vi "Interpolate_Calib_Coeff.vi"(5 "Analysis Info cluster":T1={"Colour"=0, "Inst type"=enum."Pitot-static tube", "Inst name"="Manometer voltage", "Symbol"="U", "Code name"="", "Extra Info"="U", "Inst Array"=enum."PWA", "Index"=0, "Voltage Index"=0, "Extra Titles"=[], "Extra Values"=[]}, 6 "Calib file":path, 7 "Take New Data?":bool) -> (0 "Calib Coeff":dbl[](array[numeric]), 1 "Calib Type Name":string, 2 "Calib file string":string, 3 "Read file":bool, 4 "Analysis Info cluster  Out":T1={"Colour"=0, "Inst type"=enum."Pitot-static tube", "Inst name"="Manometer voltage", "Symbol"="U", "Code name"="", "Extra Info"="U", "Inst Array"=enum."PWA", "Index"=0, "Voltage Index"=0, "Extra Titles"=[], "Extra Values"=[]})   [LabVIEW 2010]
uses:
  Controls/Analysis_info_cluster.ctl
  Controls/Inst_type.ctl
  Controls/Instrument_Array.ctl
  XW calib map/Map method.ctl
  Globals/Meas_global.vi
  XW calib map/XW_Map_Global.vi
  Globals/Plug_in_data_global.vi
  <vilib>/Analysis/NI_AALPro.lvlib
panel:
  in  "TAKE NEW DATA XW Map method":T4=enum."Const. Psi_eff (std.)"
  in  "Domain padding factor":dbl=1.01
  in  "cap indicial sum to n":bool=TRUE
  in  "surface order (n)":i32=5
  in  "Apply calibration corrections":bool=TRUE
  in  "POST PROC. XW Map method":T4=enum."Psi_eff, k = f(Umagn.)"
  in  "variable n":bool=TRUE
  in  "wire diameter (mu.m)":dbl=5.0
  out "Header info":string[][](array[string])
  # "For polysurface method only:"
  # "For trimesh method only"
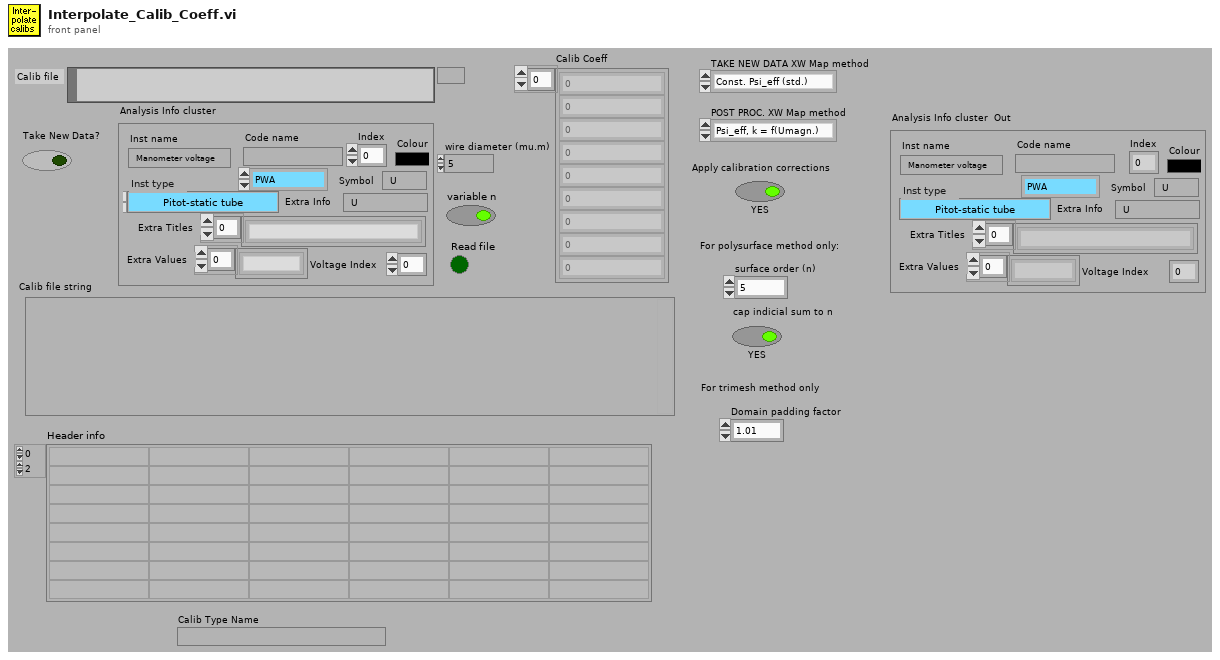
[diagram p1: front panel]
types:
  T1 = typedef "Analysis_info_cluster.ctl" = cluster{"Colour":u32, "Inst type":T2, "Inst name":string, "Symbol":string, "Code name":string, "Extra Info":string, "Inst Array":T3, "Index":i32, "Voltage Index":i32, "Extra Titles":string[], "Extra Values":string[]}
  T2 = typedef "Inst_type.ctl" = enum16{"Propeller anemometer", "Raw voltage", "Pressure Transducer", "Pitot-static tube", "Preston tube", "Hot wire", "Cross wire 1", "Cross wire 2", "Generic Linear", "Generic Polynomial", "Generic BackPoly", "Fast FID", "Thermocouple", "Cold wire", "Pulsed Wire", "LDA Vel", "LDA Tran time", "LDA Arr time"}
  T3 = typedef "Instrument_Array.ctl" = enum16{"PWA", "LDA", "Analogue"}
  T4 = typedef "Map method.ctl" = enum16{"Triangle mesh", "Polynomial surface", "Const. Psi_eff (std.)", "Psi_eff = f(Umagn.)", "Psi_eff, k = f(Umagn.)"}
  T5 = cluster{"1st Calib time":dbl, "2nd Calib time":dbl, "Meas start time":dbl, "Meas end time":dbl, "Fraction":dbl}
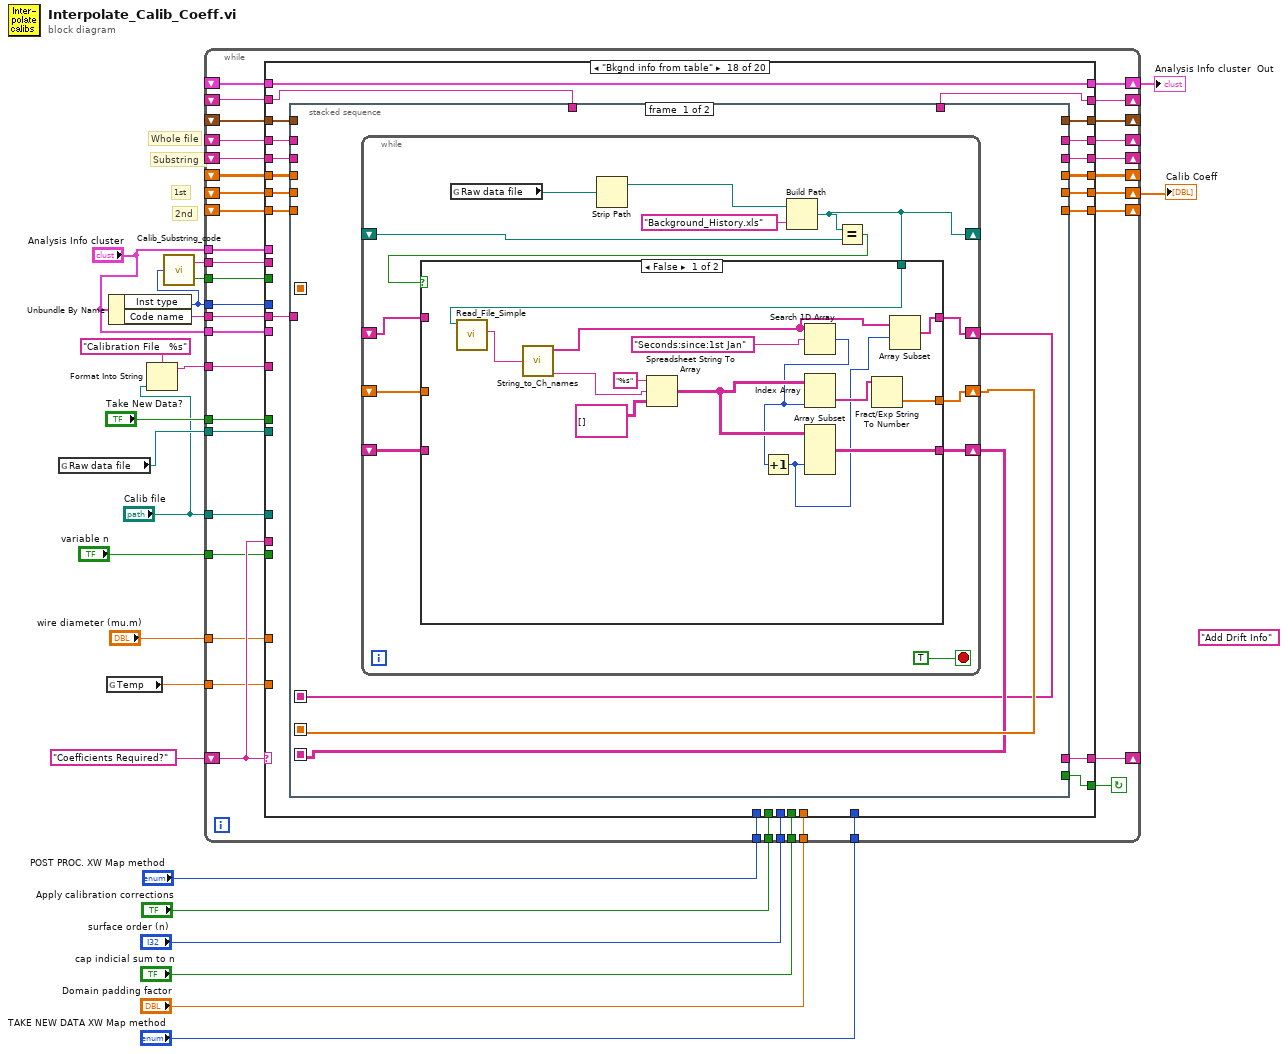
[diagram p0: block diagram]
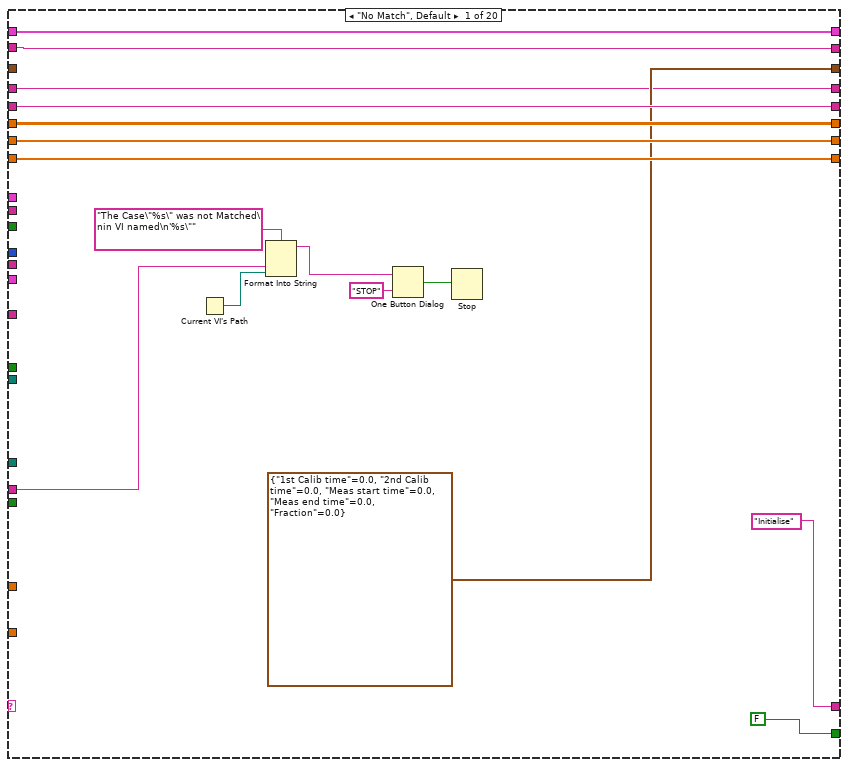
[diagram p2: hidden frame]
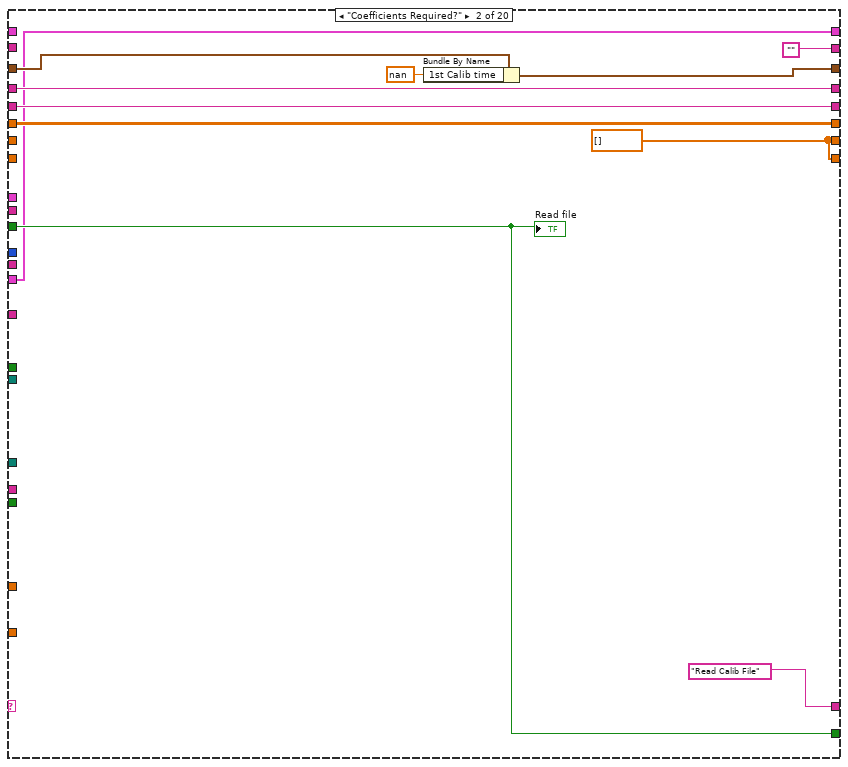
[diagram p3: hidden frame]
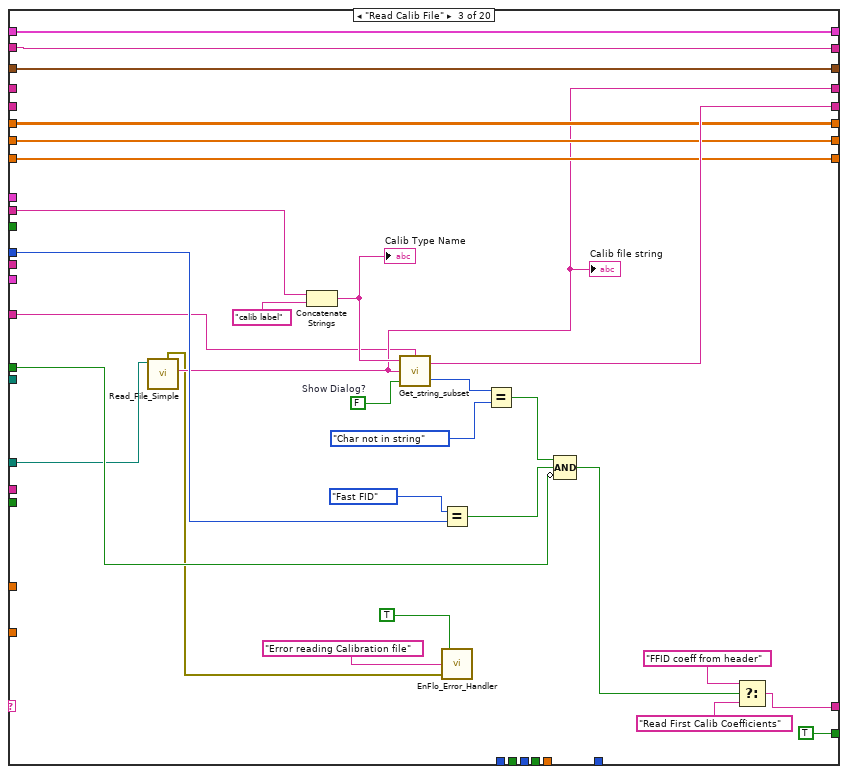
[diagram p4: hidden frame]
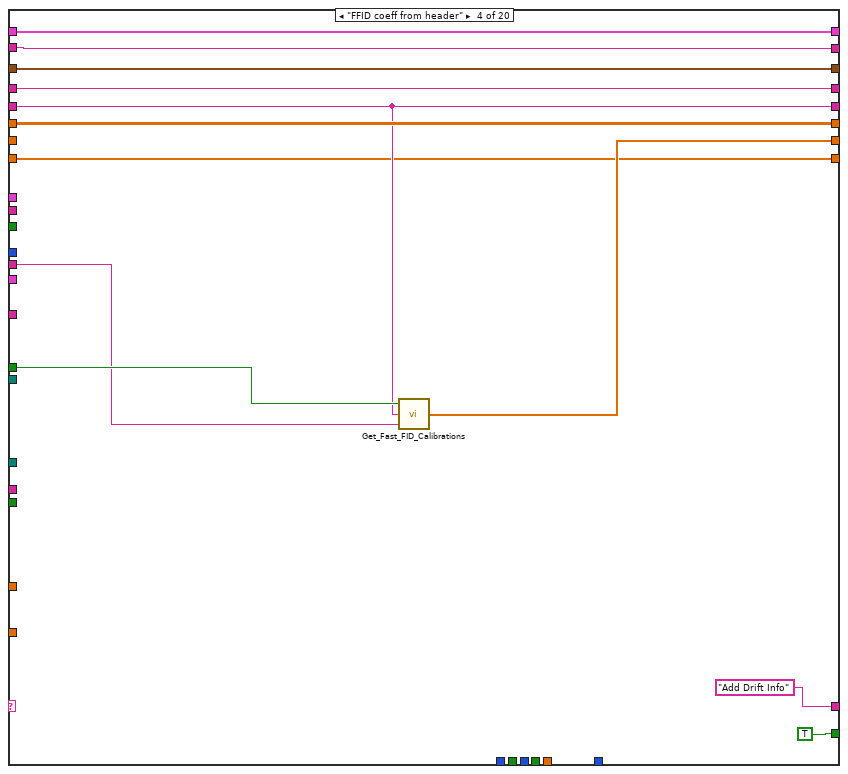
[diagram p5: hidden frame]
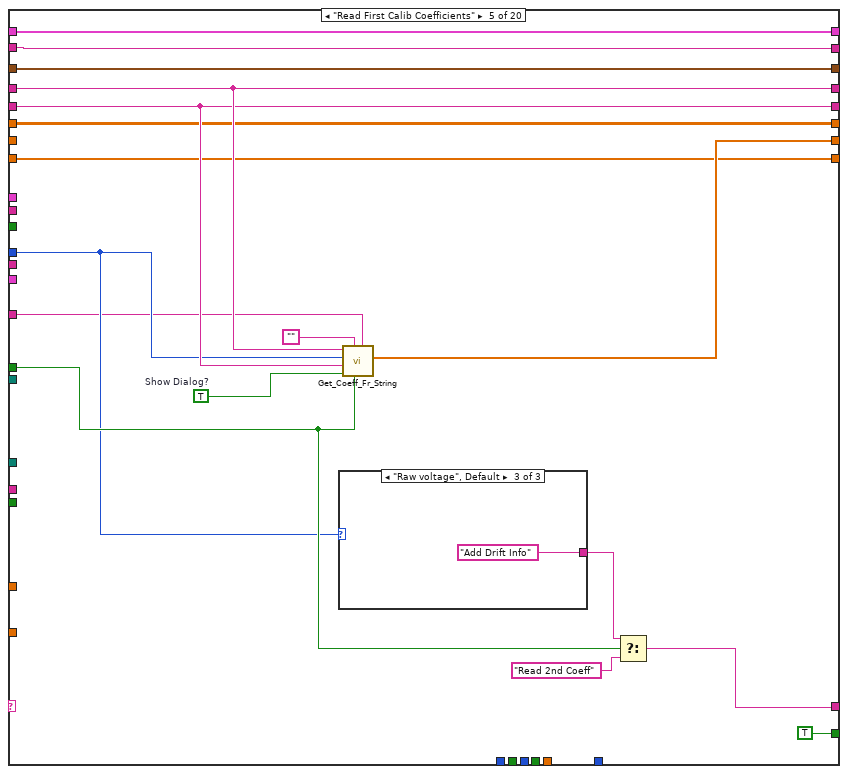
[diagram p6: hidden frame]
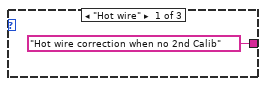
[diagram p7: hidden frame]
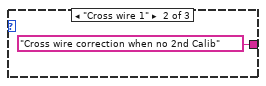
[diagram p8: hidden frame]
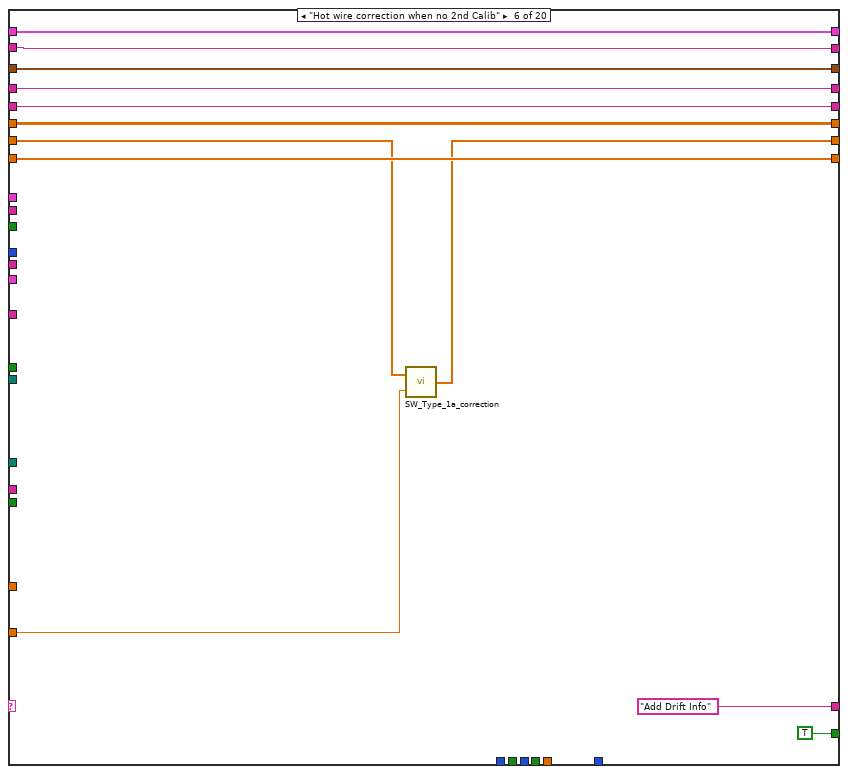
[diagram p9: hidden frame]
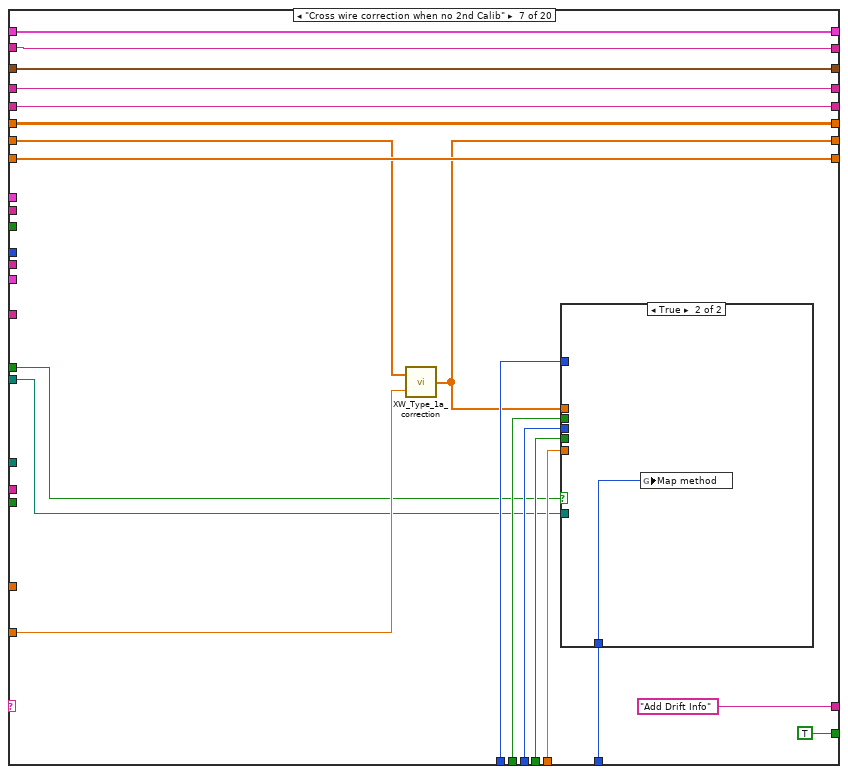
[diagram p10: hidden frame]
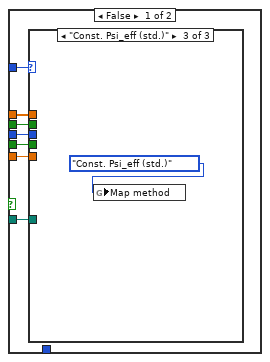
[diagram p11: hidden frame]
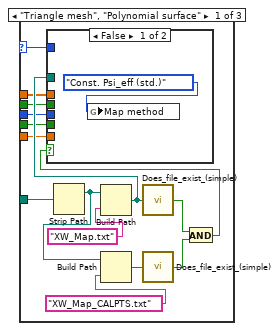
[diagram p12: hidden frame]
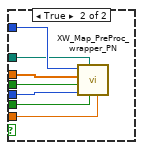
[diagram p13: hidden frame]
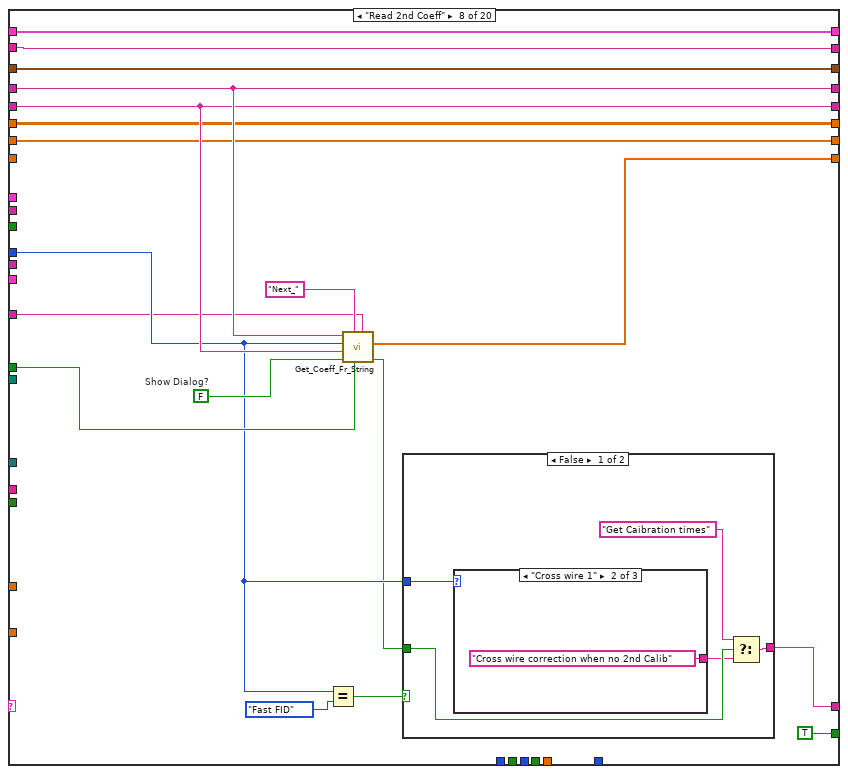
[diagram p15: hidden frame]
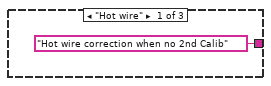
[diagram p16: hidden frame]
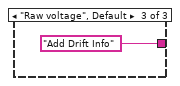
[diagram p17: hidden frame]
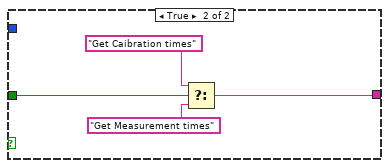
[diagram p18: hidden frame]
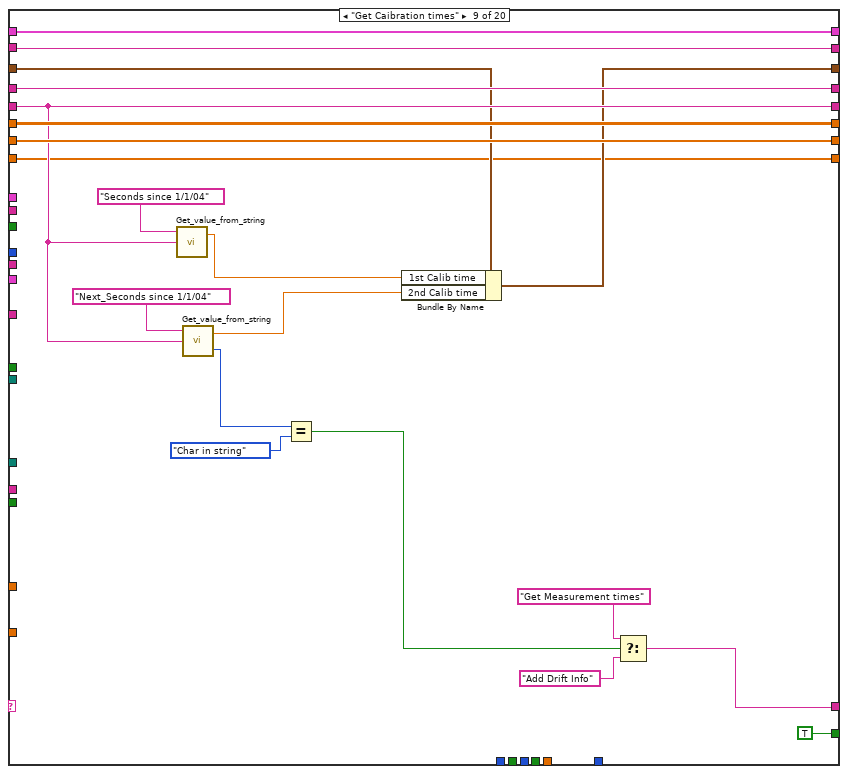
[diagram p19: hidden frame]
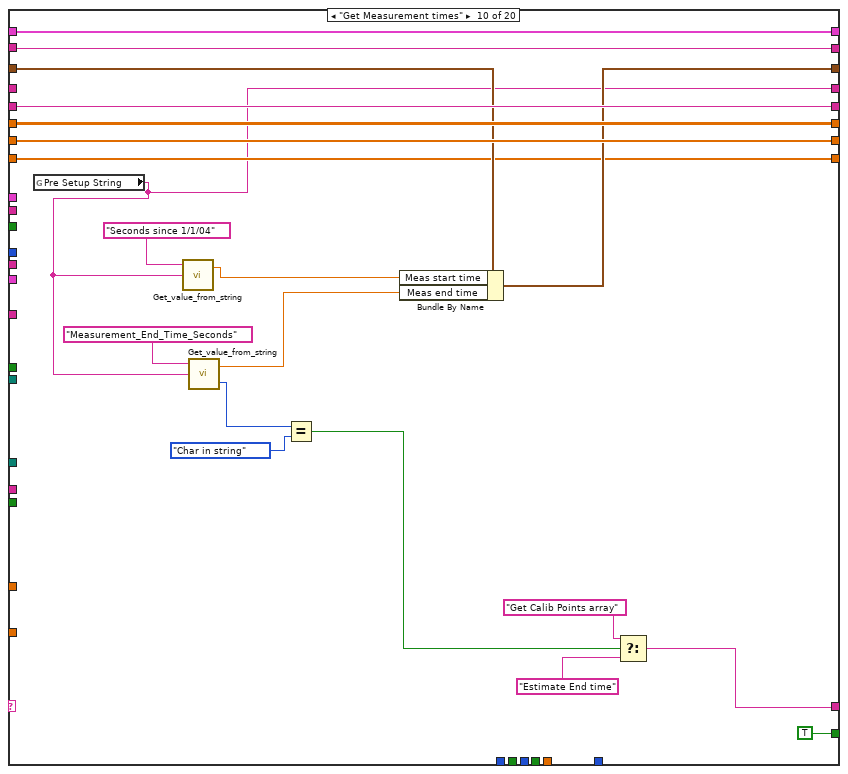
[diagram p20: hidden frame]
diagram:
  (unwired) "Add Drift Info"
  # "Substring"
  # "2nd"
  # "Whole file"
  # "1st"
  n1 = global read "Meas_global.vi" "Raw data file"() -> (w15:path)
  n2 = global read "Meas_global.vi" "Temp"() -> (w14:dbl)
  n3 = Unbundle By Name("Analysis Info cluster") -> ("Inst type"=w18:T2, "Code name"=w19:string)
  n4 = Format Into String(format string="Calibration File   %s", "Calib file") -> (resulting string=w1:string)  [unwired: 2 in, 1 out]
  n5 = call "Calib_Substring_code.vi"("Inst type"=w18) -> ("Substring Type"=w16:string, "Read file"=w17:bool)
  n6 = while {
    tunnel: "Calib file" -> [w51]
    shift-left: _ -> [w52]
    shift-right: [w53] -> _
    shift-left: _ -> [w54]
    shift-right: [w56] -> w21
    tunnel: w18 -> [w58]
    shift-left: _ -> [w55]
    shift-right: [w57] -> _
    shift-left: "Coefficients Required?" -> [w59]
    shift-right: [w24] -> _
    tunnel: "Take New Data?" -> [w50]
    tunnel: w19 -> [w49]
    shift-right: [w48] -> _
    shift-left: _ -> [w47]
    shift-right: [w46] -> _
    shift-left: _ -> [w45]
    shift-right: [w44] -> _
    shift-left: _ -> [w43]
    tunnel: w17 -> [w42]
    tunnel: w16 -> [w41]
    tunnel: w15 -> [w40]
    shift-right: [w39] -> _
    shift-left: _ -> [w38]
    tunnel: w14 -> [w37]
    tunnel: "wire diameter (mu.m)" -> [w36]
    tunnel: "variable n" -> [w35]
    tunnel: "POST PROC. XW Map method" -> [w34]
    tunnel: "Apply calibration corrections" -> [w33]
    tunnel: "surface order (n)" -> [w32]
    tunnel: "cap indicial sum to n" -> [w31]
    tunnel: "Domain padding factor" -> [w30]
    tunnel: "TAKE NEW DATA XW Map method" -> [w29]
    tunnel: "Analysis Info cluster" -> [w28]
    shift-right: [w26] -> w5
    shift-left: _ -> [w27]
    tunnel: "Analysis Info cluster" -> [w25]
    tunnel: w1 -> [w23]
    stop <- w60 continue-if-true
    n7 = case shown="\"Bkgnd info from table\"" w59 {
      tunnel: [FALSE w82 TRUE ("Read file") TRUE TRUE ("Read file") TRUE ("Read file") TRUE ("Read file") TRUE ("Read file") TRUE ("Read file") TRUE ("Read file") TRUE ("Read file") TRUE ("Read file") TRUE ("Read file") TRUE ("Read file") TRUE ("Read file") TRUE ("Read file") w507 w698 TRUE ("Read file") FALSE ("Read file")] -> w60
      tunnel: ["Initialise" "Read Calib File" w102 "Add Drift Info" w132 "Add Drift Info" "Add Drift Info" w224 w259 w280 w288 w326 "FFID Bkgnd correction method" ("f") "Add Drift Info" ("f") "Add Drift Info" ("f") w492 w508 w699 "Add Drift Info" "End"] -> w24
      tunnel: w59 -> [w71 _ _ _ _ _ _ _ _ _ _ _ _ _ _ _ _ _ _ _]
      tunnel: w58 -> [_ _ w109 _ w134 _ _ w216 _ _ _ w312 _ _ _ _ _ _ _ _]
      tunnel: [w68 w86 w115 w124 w142 w159 w179 w228 w253 w274 w305 w330 w365 w398 w444 w502 w515 w706 w804 w833] -> w57
      tunnel: [w67 w84 w99 w122 w144 w151 w162 w222 w258 w279 w306 w329 w355 w397 w404 w490 w511 w702 w795 w827] -> w56
      tunnel: w55 -> [w68 w86 _ w124 w142 w159 w179 w228 w253 w274 w305 w330 w365 w398 w444 w502 w516 w707 w804 w833]
      tunnel: w54 -> [w67 _ w99 _ _ w152 w170 w222 w258 w279 w306 w329 w356 w384 w428 w490 w512 w703 w796 w842]
      tunnel: [w66 w85 w114 w128 w141 w158 w178 w227 w261 w282 w308 w328 w351 w380 w418 w498 w514 w705 w800 w851] -> w53
      tunnel: w52 -> [w66 w85 w114 w128 w141 w158 w178 w227 w261 w282 w308 _ w351 w380 w418 w498 w513 w704 w800 w851]
      tunnel: w51 -> [_ _ w89 _ _ _ _ _ _ _ _ _ _ _ _ _ _ _ _ _]
      tunnel: w50 -> [_ _ w105 w125 w138 _ w165 w225 _ _ _ _ _ _ w406 _ _ _ _ w825]
      tunnel: w49 -> [_ _ _ w123 _ _ _ _ _ _ _ _ _ _ _ _ w519 w710 _ _]
      tunnel: [w65 w84 w98 w121 w140 w157 w177 w221 w245 w266 w303 w313 w358 w383 w429 w501 w510 w701 w803 w850] -> w48
      tunnel: w47 -> [w65 _ w98 w121 w140 w157 w177 _ w245 w266 w303 w313 w358 w383 w429 w501 w509 w700 w803 w850]
      tunnel: [w63 w83 w97 w119 w143 w160 w180 w229 w262 w265 w302 w325 w352 w394 w441 w499 w517 w708 w801 w852] -> w46
      tunnel: w45 -> [w63 w83 _ w119 w143 w160 w180 w229 w262 _ w302 w325 w352 w394 w441 w499 w520 w711 w801 w852]
      tunnel: [T5 {"1st Calib time"=0.0, "2nd Calib time"=0.0, "Meas start time"=0.0, "Meas end time"=0.0, "Fraction"=0.0} w80 w96 w120 w137 w155 w175 w220 w249 w270 w304 w314 w353 w395 w442 w500 w506 w697 w802 w830] -> w44
      tunnel: w43 -> [_ w81 w96 w120 w137 w155 w175 w220 w252 w273 w301 w316 w353 w395 w442 w500 w518 w709 w802 w830]
      tunnel: w42 -> [_ w82 _ _ _ _ _ _ _ _ _ _ _ _ _ _ _ _ _ _]
      tunnel: w41 -> [_ _ w95 _ _ _ _ _ _ _ _ _ _ _ _ _ _ _ _ _]
      tunnel: w40 -> [_ _ _ _ _ _ w164 _ _ _ w286 _ _ _ w407 w491 _ _ _ w826]
      tunnel: [w62 "" w94 w118 w135 w154 w174 w217 w244 w264 w287 w310 w342 w386 w433 w489 w505 w695 w792 w829] -> w39
      tunnel: w38 -> [w62 _ w94 w118 w135 w154 w174 w217 w244 w264 w287 w310 w344 w388 w435 w489 w504 w696 w793 w829]
      tunnel: w37 -> [_ _ _ _ _ w150 w172 _ _ _ _ _ _ w375 w409 _ _ _ _ _]
      tunnel: w36 -> [_ _ _ _ _ _ _ _ _ _ _ _ _ w373 w408 _ _ _ _ _]
      tunnel: w35 -> [_ _ _ _ _ _ _ _ _ _ _ _ _ w374 w410 _ _ _ _ _]
      tunnel: w34 -> [_ _ _ _ _ _ w171 _ _ _ _ _ _ _ w405 _ _ _ _ w824]
      tunnel: w33 -> [_ _ _ _ _ _ w169 _ _ _ _ _ _ _ w403 _ _ _ _ _]
      tunnel: w32 -> [_ _ _ _ _ _ w168 _ _ _ _ _ _ _ w402 _ _ _ _ _]
      tunnel: w31 -> [_ _ _ _ _ _ w167 _ _ _ _ _ _ _ w401 _ _ _ _ _]
      tunnel: w30 -> [_ _ _ _ _ _ w166 _ _ _ _ _ _ _ w400 _ _ _ _ _]
      tunnel: w29 -> [_ _ _ _ _ _ w163 _ _ _ _ _ _ _ _ _ _ _ _ _]
      tunnel: w28 -> [_ w77 _ _ _ _ _ _ _ _ _ _ _ _ _ _ _ _ _ w823]
      tunnel: w27 -> [w61 _ w90 w117 w131 w149 w161 w214 w243 w263 w283 w309 w341 w372 w399 w488 w503 w694 w791 _]
      tunnel: [w61 w77 w90 w117 w131 w149 w161 w214 w243 w263 w283 w309 w341 w372 w399 w488 w503 w694 w791 w822] -> w26
      tunnel: w25 -> [_ _ _ _ _ _ _ _ _ _ _ _ _ _ _ _ _ _ _ _]
      tunnel: w23 -> [_ _ w88 _ w130 _ _ w213 _ _ _ _ _ _ _ _ _ _ _ _]
      frame "No Match", Default {
        n8 = Current VI's Path() -> (path=w70:path)
        n9 = Format Into String(format string="The Case\"%s\" was not Matched\nin VI named\n'%s\"" ("Format String"), w71, w70) -> (resulting string=w74:string)  [unwired: 2 in, 1 out]
        n10 = One Button Dialog(message=w74, button name ("OK")="STOP") -> (true=w72:bool)
        n11 = Stop(stop? (T)=w72) -> ()
      }
      frame "Coefficients Required?" {
        w84 = dbl[] [] ("Calib Coeff")
        n12 = Bundle By Name(cluster=w81, "1st Calib time"=nan) -> (w80:T5)
        "Read file" <- w82
      }
      frame "Read Calib File" {
        w110 = FALSE  # Show Dialog?
        n13 = call "Read_File_Simple.vi"("Filename"=w89) -> ("error out"=w93:errorcluster, "string"=w97:string)  [unwired: 2 in, 6 out]
        "Calib file string" <- w97
        n14 = Concatenate Strings(w95, "calib label") -> (w113:string)
        "Calib Type Name" <- w113
        n15 = call "Get_string_subset.vi"("String Name"=w88, "Show Dialog?"=w110, "String to split"=w97, "File Label"=w113) -> ("Status"=w112:enum16{"Char in string", "Char not in string"}, "Output string"=w115:string)
        n16 = Equal?(x=Inst_type."Fast FID" ("Inst type"), y=w109) -> (x = y?=w106:bool)
        n17 = call "EnFlo_Error_Handler.vi"("error in (no error)"=w93, "Error Type"="Error reading Calibration file", "Dialog Box (T)"=TRUE) -> ()  [unwired: 3 out]
        n18 = Equal?(x=w112, y=enum16{"Char in string", "Char not in string"}."Char not in string" ("Status")) -> (x = y?=w107:bool)
        n19 = Compound Arithmetic op=AND(w107, w106, invert w105) -> (w103:bool)
        n20 = Select(t="FFID coeff from header", s=w103, f="Read First Calib Coefficients") -> (s? t:f=w102:string)
      }
      frame "FFID coeff from header" {
        n21 = call "Get_Fast_FID_Calibrations.vi"("Code Name"=w123, "Calib File String"=w124, "Take New Data"=w125) -> ("Calib Constants"=w122:dbl[])
      }
      frame "Read First Calib Coefficients" {
        w145 = TRUE  # Show Dialog?
        n22 = case shown="\"Raw voltage\", Default" w134 {
          tunnel: ["Hot wire correction when no 2nd Calib" "Cross wire correction when no 2nd Calib" "Add Drift Info"] -> w133
          frame "Hot wire" {
          }
          frame "Cross wire 1" {
          }
          frame "Raw voltage", Default {
          }
        }
        n23 = call "Get_Coeff_Fr_String.vi"("String Name"=w130, "Take New Data?"=w138, "Prefix"="", "Show Dialog?"=w145, "Sub String"=w142, "Inst type"=w134, "Whole String"=w143) -> ("Calib Constants"=w144:dbl[])  [unwired: 2 in, 1 out]
        n24 = Select(t=w133, s=w138, f="Read 2nd Coeff") -> (s? t:f=w132:string)
      }
      frame "Hot wire correction when no 2nd Calib" {
        n25 = call "SW_Type_1a_correction.vi"("Tmeas (degC)"=w150, "Calib consts."=w152) -> ("Corrected calib consts."=w151:dbl[])
      }
      frame "Cross wire correction when no 2nd Calib" {
        n26 = call "XW_Type_1a_correction.vi"("Tmeas (degC)"=w172, "Calib consts."=w170) -> ("Corrected calib consts."=w162:dbl[])
        n27 = case shown="True" w165 {
          tunnel: w164 -> [w187 _]
          tunnel: w171 -> [w181 _]
          tunnel: w162 -> [w186 _]
          tunnel: w169 -> [w185 _]
          tunnel: w168 -> [w184 _]
          tunnel: w167 -> [w183 _]
          tunnel: w166 -> [w182 _]
          tunnel: w163 -> [_ w212]
          frame False {
            n28 = case shown="\"Const. Psi_eff (std.)\"" w181 {
              selector: w181 -> [w194 _ _]
              tunnel: w187 -> [w202 _ _]
              tunnel: w186 -> [w199 _ _]
              tunnel: w185 -> [w198 _ _]
              tunnel: w184 -> [w197 _ _]
              tunnel: w183 -> [w196 _ _]
              tunnel: w182 -> [w195 _ _]
              frame "Triangle mesh", "Polynomial surface" {
                n29 = Strip Path(path=w202) -> (stripped path=w191:path)  [unwired: 1 out]
                n30 = Build Path(base path=w191, name or relative path="XW_Map.txt") -> (appended path=w200:path)
                n31 = Build Path(base path=w191, name or relative path="XW_Map_CALPTS.txt") -> (appended path=w193:path)
                n32 = call "Does_file_exist_(simple).vi"("Pathname"=w200) -> ("exists?"=w189:bool)
                n33 = call "Does_file_exist_(simple).vi"("Pathname"=w193) -> ("exists?"=w190:bool)
                n34 = And(x=w189, y=w190) -> (x .and. y?=w188:bool)
                n35 = case shown="False" w188 {
                  tunnel: w200 -> [_ w209]
                  tunnel: w194 -> [_ w210]
                  tunnel: w199 -> [_ w208]
                  tunnel: w198 -> [_ w207]
                  tunnel: w197 -> [_ w206]
                  tunnel: w196 -> [_ w205]
                  tunnel: w195 -> [_ w204]
                  frame False {
                    n36 = global write "XW_Map_Global.vi" "Map method"(Map_method."Const. Psi_eff (std.)" ("Map method")) -> ()
                  }
                  frame True {
                    n37 = call "XW_Map_PreProc_wrapper_PN.vi"("Domain padding factor"=w204, "cap indicial sum to n"=w205, "XW_Calib_Map file path"=w209, "surface order (n)"=w206, "Apply calibration corrections"=w207, "Calib const"=w208, "Map method"=w210) -> ()  [unwired: 5 out]
                  }
                }
              }
              frame "Psi_eff = f(Umagn.)", "Psi_eff, k = f(Umagn.)" {
              }
              frame "Const. Psi_eff (std.)" {
                n38 = global write "XW_Map_Global.vi" "Map method"(Map_method."Const. Psi_eff (std.)" ("Map method")) -> ()
              }
            }
          }
          frame True {
            n39 = global write "XW_Map_Global.vi" "Map method"(w212) -> ()
          }
        }
      }
      frame "Read 2nd Coeff" {
        w230 = FALSE  # Show Dialog?
        n40 = Equal?(x=w216, y=Inst_type."Fast FID" ("Inst type")) -> (x = y?=w218:bool)
        n41 = call "Get_Coeff_Fr_String.vi"("String Name"=w213, "Take New Data?"=w225, "Prefix"="Next_", "Show Dialog?"=w230, "Sub String"=w228, "Inst type"=w216, "Whole String"=w229) -> ("Coefficients Found?"=w215:bool, "Calib Constants"=w221:dbl[])  [unwired: 2 in]
        n42 = case shown="False" w218 {
          tunnel: [w231 w242] -> w224
          tunnel: w215 -> [w233 w239]
          tunnel: w216 -> [w235 _]
          frame False {
            n43 = case shown="\"Cross wire 1\"" w235 {
              tunnel: ["Hot wire correction when no 2nd Calib" "Cross wire correction when no 2nd Calib" "Add Drift Info"] -> w232
              frame "Hot wire" {
              }
              frame "Cross wire 1" {
              }
              frame "Raw voltage", Default {
              }
            }
            n44 = Select(t="Get Caibration times", s=w233, f=w232) -> (s? t:f=w231:string)
          }
          frame True {
            n45 = Select(t="Get Caibration times", s=w239, f="Get Measurement times") -> (s? t:f=w242:string)
          }
        }
      }
      frame "Get Caibration times" {
        n46 = call "Get_value_from_string.vi"("Input string"=w253, "Variable name"="Seconds since 1/1/04") -> ("Value"=w251:dbl)  [unwired: 1 in, 1 out]
        n47 = call "Get_value_from_string.vi"("Input string"=w253, "Variable name"="Next_Seconds since 1/1/04") -> ("Status"=w248:enum16{"Char in string", "Char not in string"}, "Value"=w250:dbl)  [unwired: 1 in]
        n48 = Equal?(x=w248, y=enum16{"Char in string", "Char not in string"}."Char in string" ("Status")) -> (x = y?=w246:bool)
        n49 = Bundle By Name(cluster=w252, "1st Calib time"=w251, "2nd Calib time"=w250) -> (w249:T5)
        n50 = Select(t="Get Measurement times", s=w246, f="Add Drift Info") -> (s? t:f=w259:string)
      }
      frame "Get Measurement times" {
        n51 = global read "Meas_global.vi" "Pre Setup String"() -> (w265:string)
        n52 = call "Get_value_from_string.vi"("Input string"=w265, "Variable name"="Seconds since 1/1/04") -> ("Value"=w272:dbl)  [unwired: 1 in, 1 out]
        n53 = call "Get_value_from_string.vi"("Input string"=w265, "Variable name"="Measurement_End_Time_Seconds") -> ("Status"=w269:enum16{"Char in string", "Char not in string"}, "Value"=w271:dbl)  [unwired: 1 in]
        n54 = Equal?(x=w269, y=enum16{"Char in string", "Char not in string"}."Char in string" ("Status")) -> (x = y?=w267:bool)
        n55 = Bundle By Name(cluster=w273, "Meas start time"=w272, "Meas end time"=w271) -> (w270:T5)
        n56 = Select(t="Get Calib Points array", s=w267, f="Estimate End time") -> (s? t:f=w280:string)
      }
      frame "Estimate End time" {
        n57 = Unbundle By Name(w301) -> ("Meas start time"=w300:dbl)
        n58 = call "Read_RD_Ch_header.vi"("Raw data file"=w286) -> ("Ch Name Out"=w285:string[], "Ch Values"=w284:string[])  [unwired: 2 out]
        n59 = Search 1D Array(1D array=w285, element="Flow:Measurement:Time") -> (index of element=w297:i32)  [unwired: 1 out]
        n60 = Index Array(array=w284, index=w297) -> (element=w296:string)
        n61 = Fract/Exp String To Number(string=w296, default (0 dbl)=nan ("default (0 DBL)")) -> (number=w292:dbl)  [unwired: 3 out]
        n62 = Not A Number/Path/Refnum?(number/path/refnum=w292) -> (NaN/Path/Refnum?=w291:bool)
        n63 = Multiply(x=w292, y=60.0) -> (x*y=w293:dbl)
        n64 = Add(x=w300, y=w293) -> (x+y=w299:dbl)
        n65 = Bundle By Name(cluster=w301, "Meas end time"=w299) -> (w304:T5)
        n66 = Select(t="Add Drift Info", s=w291, f="Get Calib Points array") -> (s? t:f=w288:string)
      }
      frame "Get Calib Points array" {
        w332 = FALSE  # Show Dialog?
        # "Fraction = (Av_Meas_Time - Calib1_time)  /  (Calib2_time - Calib1_time)"
        n67 = Unbundle By Name(w316) -> ("Meas start time"=w321:dbl, "Meas end time"=w320:dbl, "2nd Calib time"=w322:dbl, "1st Calib time"=w311:dbl)
        n68 = Add(x=w321, y=w320) -> (x+y=w324:dbl)
        n69 = call "2D_array_from_string.vi"("Show Dialog?"=w332, "Input string"=w330, "Array title"="Calib points label") -> ("2D data array"=w328:dbl[][])  [unwired: 1 in]
        n70 = Divide(x=w324, y=2.0) -> (x/y=w319:dbl)
        n71 = Subtract(x=w322, y=w311) -> (x-y=w317:dbl)
        n72 = Subtract(x=w319, y=w311) -> (x-y=w318:dbl)
        n73 = Divide(x=w318, y=w317) -> (x/y=w315:dbl)
        n74 = case shown="\"Hot wire\"" w312 {
          tunnel: ["Add Drift Info" "Single Hot wire" "Cross wire" w337] -> w326
          tunnel: w311 -> [_ _ _ w340]
          frame "Propeller anemometer", Default {
          }
          frame "Hot wire" {
          }
          frame "Cross wire 1" {
          }
          frame "Fast FID" {
            n75 = Not A Number/Path/Refnum?(number/path/refnum=w340) -> (NaN/Path/Refnum?=w339:bool)
            n76 = Select(t="FFID Bkgnd correction method", s=w339, f="Fast FID") -> (s? t:f=w337:string)
          }
        }
        n77 = Bundle By Name(cluster=w316, "Fraction"=w315) -> (w314:T5)
      }
      frame "Fast FID" {
        # "Concentrations"
        # "Voltage"
        # "End"
        # "Start"
        # "(End-Start)*Fraction + Start"
        n78 = Index Array(array=w351, index (col)=1) -> (element=w361:dbl[])  [unwired: 1 in]
        n79 = call "2nd_order_Poly_convert.vi"("Calib constants"=w358, "Voltage"=w361) -> ("Eng Values"=w362:dbl[])  [unwired: 4 out]
        n80 = call "2nd_order_Poly_convert.vi"("Calib constants"=w356, "Voltage"=w361) -> ("Eng Values"=w363:dbl[])  [unwired: 4 out]
        n81 = Unbundle By Name(w353) -> ("Fraction"=w348:dbl)
        n82 = In Range and Coerce(upper limit=1.0, x=w348, lower limit=0.0) -> (coerced(x)=w345:dbl)  [unwired: 1 out]
        n83 = for {
          tunnel: w363 -> [w367] mode=indexing
          tunnel: w362 -> [w371] mode=indexing
          tunnel: w345 -> [w369]
          tunnel: [w366] -> w360 mode=indexing
          n84 = Subtract(x=w371, y=w367) -> (x-y=w370:dbl)
          n85 = Multiply(x=w369, y=w370) -> (x*y=w368:dbl)
          n86 = Add(x=w367, y=w368) -> (x+y=w366:dbl)
        }
        n87 = Format Into String(format string="Calib Fraction %.4f; ", initial string=w344, w345) -> (resulting string=w342:string)  [unwired: 1 in, 1 out]
        n88 = call <vilib>:"General Polynomial Fit.vi"("Y"=w360, "polynomial order"=2, "X"=w361) -> ("Polynomial Coefficients"=w357:dbl[])  [unwired: 9 in, 3 out]
        n89 = Replace Array Subset(array=w356, new element=w357, index=0) -> (w355:dbl[])
      }
      frame "Single Hot wire" {
        n90 = Index Array(array=w380, index (col)=1) -> (element=w379:dbl[])  [unwired: 1 in]
        n91 = Index Array(array=w380, index (col)=0) -> (element=w378:dbl[])  [unwired: 1 in]
        n92 = Unbundle By Name(w395) -> ("Fraction"=w391:dbl)
        n93 = In Range and Coerce(upper limit=1.0, x=w391, lower limit=0.0) -> (coerced(x)=w377:dbl)  [unwired: 1 out]
        n94 = call "SingleWire_drift_correction_PN.vi"("calib consts. t1"=w384, "Tmeas (degC)"=w375, "variable n"=w374, "calib consts. t2"=w383, "{E_cal1}"=w379, "{U_cal1}"=w378, "time fraction"=w377, "wire diameter (mu.m)"=w373) -> ("[A, B, n]"=w376:dbl[])  [unwired: 1 in, 6 out]
        n95 = Build Array (concatenate)(w376, w375) -> (w385:dbl[])
        n96 = Format Into String(format string="Calib Fraction %.4f; ", initial string=w388, w377) -> (resulting string=w386:string)  [unwired: 1 in, 1 out]
        n97 = Replace Array Subset(array=w384, new element=w385, index=0) -> (w397:dbl[])
      }
      frame "Cross wire" {
        n98 = for {
          tunnel: w428 -> [w485]
          tunnel: w429 -> [w484]
          tunnel: [w483] -> w422 mode=indexing
          tunnel: [w482] -> w421 mode=indexing
          tunnel: i32[] [0, 1, 2, 9, 10, 12, 14, 15] -> [w481] mode=indexing
          n99 = Index Array(array=w485, index=w481) -> (element=w483:dbl)
          n100 = Index Array(array=w484, index=w481) -> (element=w482:dbl)
        }
        n101 = for {
          tunnel: i32[] [3, 4, 5, 9, 11, 13, 16, 17] -> [w480] mode=indexing
          tunnel: w429 -> [w479]
          tunnel: [w478] -> w414 mode=indexing
          tunnel: w428 -> [w477]
          tunnel: [w476] -> w415 mode=indexing
          n102 = Index Array(array=w477, index=w480) -> (element=w476:dbl)
          n103 = Index Array(array=w479, index=w480) -> (element=w478:dbl)
        }
        n104 = Index Array(array=w418, index (col)=1) -> (element=w420:dbl[])  [unwired: 1 in]
        n105 = Index Array(array=w418, index (col)=0) -> (element=w417:dbl[])  [unwired: 1 in]
        n106 = Index Array(array=w418, index (col)=2) -> (element=w416:dbl[])  [unwired: 1 in]
        n107 = Unbundle By Name(w442) -> ("Fraction"=w438:dbl)
        n108 = In Range and Coerce(upper limit=1.0, x=w438, lower limit=0.0) -> (coerced(x)=w413:dbl)  [unwired: 1 out]
        n109 = call "SingleWire_drift_correction_PN.vi"("calib consts. t1"=w422, "Tmeas (degC)"=w409, "variable n"=w410, "calib consts. t2"=w421, "{E_cal1}"=w420, "{U_cal1}"=w417, "time fraction"=w413, "wire diameter (mu.m)"=w408) -> ("[A, B, n]"=w412:dbl[])  [unwired: 1 in, 6 out]
        n110 = call "SingleWire_drift_correction_PN.vi"("calib consts. t1"=w415, "Tmeas (degC)"=w409, "variable n"=w410, "calib consts. t2"=w414, "{E_cal1}"=w416, "{U_cal1}"=w417, "time fraction"=w413, "wire diameter (mu.m)"=w408) -> ("[A, B, n]"=w411:dbl[])  [unwired: 1 in, 6 out]
        n111 = Replace Array Subset(array=w428, new element=w409, index=9) -> (w424:dbl[])
        n112 = Replace Array Subset(array=w424, new element=w412, index=0) -> (w423:dbl[])
        n113 = Replace Array Subset(array=w423, new element=w411, index=3) -> (w404:dbl[])
        n114 = Format Into String(format string="Calib Fraction %.4f; ", initial string=w435, w413) -> (resulting string=w433:string)  [unwired: 1 in, 1 out]
        n115 = case shown="False" w406 {
          tunnel: w407 -> [w451 _]
          tunnel: w405 -> [w445 _]
          tunnel: w404 -> [w450 _]
          tunnel: w403 -> [w449 _]
          tunnel: w402 -> [w448 _]
          tunnel: w401 -> [w447 _]
          tunnel: w400 -> [w446 _]
          frame False {
            n116 = case shown="\"Triangle mesh\", \"Polynomial surface\"" w445 {
              selector: w445 -> [w458 _ _]
              tunnel: w451 -> [w466 _ _]
              tunnel: w450 -> [w463 _ _]
              tunnel: w449 -> [w462 _ _]
              tunnel: w448 -> [w461 _ _]
              tunnel: w447 -> [w460 _ _]
              tunnel: w446 -> [w459 _ _]
              frame "Triangle mesh", "Polynomial surface" {
                n117 = Strip Path(path=w466) -> (stripped path=w455:path)  [unwired: 1 out]
                n118 = Build Path(base path=w455, name or relative path="XW_Map.txt") -> (appended path=w464:path)
                n119 = Build Path(base path=w455, name or relative path="XW_Map_CALPTS.txt") -> (appended path=w457:path)
                n120 = call "Does_file_exist_(simple).vi"("Pathname"=w464) -> ("exists?"=w453:bool)
                n121 = call "Does_file_exist_(simple).vi"("Pathname"=w457) -> ("exists?"=w454:bool)
                n122 = And(x=w453, y=w454) -> (x .and. y?=w452:bool)
                n123 = case shown="False" w452 {
                  tunnel: w464 -> [_ w473]
                  tunnel: w458 -> [_ w474]
                  tunnel: w463 -> [_ w472]
                  tunnel: w462 -> [_ w471]
                  tunnel: w461 -> [_ w470]
                  tunnel: w460 -> [_ w469]
                  tunnel: w459 -> [_ w468]
                  frame False {
                    n124 = global write "XW_Map_Global.vi" "Map method"(Map_method."Const. Psi_eff (std.)" ("Map method")) -> ()
                  }
                  frame True {
                    n125 = call "XW_Map_PreProc_wrapper_PN.vi"("Domain padding factor"=w468, "cap indicial sum to n"=w469, "XW_Calib_Map file path"=w473, "surface order (n)"=w470, "Apply calibration corrections"=w471, "Calib const"=w472, "Map method"=w474) -> ()  [unwired: 5 out]
                  }
                }
              }
              frame "Psi_eff = f(Umagn.)", "Psi_eff, k = f(Umagn.)" {
              }
              frame "Const. Psi_eff (std.)" {
                n126 = global write "XW_Map_Global.vi" "Map method"(Map_method."Const. Psi_eff (std.)" ("Map method")) -> ()
              }
            }
          }
          frame True {
          }
        }
      }
      frame "FFID Bkgnd correction method" {
        n127 = Strip Path(path=w491) -> (stripped path=w495:path)  [unwired: 1 out]
        n128 = Build Path(base path=w495, name or relative path="Background_History.xls") -> (appended path=w494:path)
        n129 = call "Does_file_exist_(simple).vi"("Pathname"=w494) -> ("exists?"=w493:bool)
        n130 = Select(t="Bkgnd info from table", s=w493, f="Bkgnd info from header") -> (s? t:f=w492:string)
      }
      frame "Bkgnd info from header" {
        n131 = stacked-sequence {
          seq-local: [w521 _ _ _] -> [_ _ w566 _]
          seq-local: [w533 _ _ _] -> [_ _ w564 _]
          seq-local: [w528 _ _ _] -> [_ _ w563 _]
          seq-local: [_ w556 _ _] -> [_ _ w562 _]
          seq-local: [_ _ w561 _] -> [_ _ _ w662]
          tunnel: w520 -> [w535 w555 _ _]
          tunnel: w519 -> [_ _ w565 _]
          tunnel: w518 -> [_ w551 _ _]
          tunnel: [_ w555 _ _] -> w517
          tunnel: w516 -> [_ w554 _ _]
          tunnel: [_ w554 _ _] -> w515
          tunnel: [_ w553 _ _] -> w514
          tunnel: w513 -> [_ w553 _ _]
          tunnel: w512 -> [_ _ _ w672]
          tunnel: [_ _ _ w669] -> w511
          tunnel: [_ w552 _ _] -> w510
          tunnel: w509 -> [_ w552 _ _]
          tunnel: [_ _ _ "Add FFID Bkgnd Values"] -> w508
          tunnel: [_ _ _ TRUE] -> w507
          tunnel: [_ w551 _ _] -> w506
          tunnel: [_ _ _ w664] -> w505
          tunnel: w504 -> [_ _ _ w663]
          frame #0 {
            n132 = Concatenate Strings("Calibration To be Used" ("Input Element"), "\t") -> (w537:string)
            n133 = Match Pattern(string=w535, regular expression=w537) -> (before substring=w542:string, match substring=w548:string, after substring=w549:string)  [unwired: 2 out]
            n134 = Reverse String(1:w542) -> (0:w543:string)
            n135 = Match Pattern(string=w543, regular expression="[*][*][*][*][*][*][*][*][*][*][*][*][*][\t][*][*][*][*][*][*][*][*][*][*][*][*][*][\t][*][*][*][*][*][*][*][*][*][*][*][*][*][\t][*][*][*][*]" ("String")) -> (before substring=w541:string)  [unwired: 4 out]
            n136 = Reverse String(1:w541) -> (0:w540:string)
            n137 = call "Split_at_return.vi"("String"=w540) -> ("after substring"=w539:string)  [unwired: 1 in, 3 out]
            n138 = call "String_to_Ch_names.vi"("Spreadsheet string"=w539) -> ("Ch names"=w533:string[], "String After names"=w547:string)  [unwired: 2 out]
            n139 = Concatenate Strings(w547, w548, w549) -> (w550:string)
            n140 = Search 1D Array(1D array=w533, element="FF:1:Bkgnd Volts") -> (index of element=w527:i32)  [unwired: 1 out]
            n141 = Spreadsheet String To Array(format string="%s", spreadsheet string=w550, array type (2D Dbl)=string[][] []) -> (array=w528:string[][])  [unwired: 1 out]
            "Header info" <- w528
            n142 = Index Array(array=w528, index (col)=0 ("disabled index (col)")) -> (element=w530:string[])  [unwired: 1 in]
            n143 = Search 1D Array(1D array=w530, element="Calibration After Meas") -> (index of element=w529:i32)  [unwired: 1 out]
            n144 = Index Array(array=w528, index (row)=w529, index (col)=w527) -> (element=w526:string)
            n145 = Match Pattern(string=w526, regular expression="_Place_Holder") -> (offset past match=w524:i32)  [unwired: 4 out]
            n146 = Less Than 0?(x=w524) -> (x < 0?=w522:bool)
            n147 = Greater Or Equal To 0?(x=w527) -> (x >= 0?=w523:bool)
            n148 = And(x=w523, y=w522) -> (x .and. y?=w521:bool)
          }
          frame #1 {
            n149 = Unbundle By Name(w551) -> ("Meas start time"=w560:dbl, "Meas end time"=w559:dbl)
            n150 = Add(x=w560, y=w559) -> (x+y=w558:dbl)
            n151 = Divide(x=w558, y=2.0) -> (x/y=w556:dbl)
          }
          frame #2 {
            n152 = case shown="False" w566 {
              tunnel: w565 -> [w582 w636]
              tunnel: w564 -> [w569 w626]
              tunnel: w563 -> [w571 w627]
              tunnel: w562 -> [w568 _]
              tunnel: [w567 w619] -> w561
              frame True {
                n153 = Decimal String To Number(string=w582) -> (number=w581:i32)  [unwired: 3 out]
                n154 = Index Array(array=w571, index (col)=0 ("disabled index (col)")) -> (element=w576:string[])  [unwired: 1 in]
                n155 = Number To Decimal String(number=w581) -> (decimal integer string=w580:string)  [unwired: 1 out]
                n156 = Search 1D Array(1D array=w576, element="Calibration Before Meas") -> (index of element=w574:i32)  [unwired: 1 out]
                n157 = Search 1D Array(1D array=w576, element="Calibration After Meas") -> (index of element=w572:i32)  [unwired: 1 out]
                n158 = Index Array(array=w571, index (row)=w574) -> (element=w573:string[])  [unwired: 1 in]
                n159 = Index Array(array=w571, index (row)=w572) -> (element=w570:string[])  [unwired: 1 in]
                n160 = for {
                  tunnel: w580 -> [w598]
                  tunnel: string[] ["Bkgnd Time", "Bkgnd Volts", "Bkgnd Variance"] ("appended array") -> [w597] mode=indexing
                  tunnel: w573 -> [w596]
                  tunnel: w570 -> [w594]
                  tunnel: w569 -> [w592]
                  tunnel: w568 -> [w590]
                  shift-right: [w584] -> _
                  shift-left: _ -> [w585]
                  tunnel: [w583] -> w567 mode=indexing
                  i -> [w591]
                  # "After"
                  # "Before"
                  n161 = Concatenate Strings("FF:", w598, ":" ("Substring"), w597) -> (w599:string)
                  n162 = Search 1D Array(1D array=w592, element=w599) -> (index of element=w595:i32)  [unwired: 1 out]
                  n163 = Index Array(array=w596, index=w595) -> (element=w589:string)
                  n164 = Index Array(array=w594, index=w595) -> (element=w588:string)
                  n165 = Fract/Exp String To Number(string=w589) -> (number=w587:dbl)  [unwired: 4 out]
                  n166 = Fract/Exp String To Number(string=w588) -> (number=w586:dbl)  [unwired: 4 out]
                  n167 = case shown="1, Default" w591 {
                    tunnel: w590 -> [w606 _]
                    tunnel: w587 -> [w604 w609]
                    tunnel: w586 -> [w605 w612]
                    tunnel: [w601 w608] -> w583
                    tunnel: w585 -> [_ w607]
                    tunnel: [w601 w607] -> w584
                    frame 0 {
                      n168 = Subtract(x=w606, y=w604) -> (x-y=w602:dbl)
                      n169 = Subtract(x=w605, y=w604) -> (x-y=w603:dbl)
                      n170 = Divide(x=w602, y=w603) -> (x/y=w601:dbl)
                    }
                    frame 1, Default {
                      n171 = Subtract(x=w612, y=w609) -> (x-y=w611:dbl)
                      n172 = Multiply(x=w607, y=w611) -> (x*y=w610:dbl)
                      n173 = Add(x=w610, y=w609) -> (x+y=w608:dbl)
                    }
                  }
                }
              }
              frame False {
                n174 = Decimal String To Number(string=w636) -> (number=w635:i32)  [unwired: 3 out]
                n175 = Index Array(array=w627, index (col)=0 ("disabled index (col)")) -> (element=w630:string[])  [unwired: 1 in]
                n176 = Number To Decimal String(number=w635) -> (decimal integer string=w634:string)  [unwired: 1 out]
                n177 = Search 1D Array(1D array=w630, element="Calibration To be Used") -> (index of element=w629:i32)  [unwired: 1 out]
                n178 = Index Array(array=w627, index (row)=w629) -> (element=w628:string[])  [unwired: 1 in]
                n179 = for {
                  tunnel: w634 -> [w657]
                  tunnel: string[] ["Coeff A", "Coeff B", "Coeff C", "Bkgnd", "Bkgnd Variance"] ("appended array") -> [w656] mode=indexing
                  tunnel: w628 -> [w655]
                  tunnel: w626 -> [w653]
                  tunnel: [w651] -> w615 mode=indexing
                  tunnel: [w650] -> w618 mode=indexing
                  n180 = Concatenate Strings("FF:", w657, ":" ("Substring"), w656) -> (w658:string)
                  n181 = Search 1D Array(1D array=w653, element=w658) -> (index of element=w650:i32)  [unwired: 1 out]
                  n182 = Index Array(array=w655, index=w650) -> (element=w652:string)
                  n183 = Fract/Exp String To Number(string=w652) -> (number=w651:dbl)  [unwired: 4 out]
                }
                n184 = Index Array(array=w615, index=3 ("length")) -> (element=w624:dbl)
                n185 = Index Array(array=w615, index=4) -> (element=w621:dbl)
                n186 = Index Array(array=w618, index=2) -> (element=w616:i32)
                n187 = Less Than 0?(x=w616) -> (x < 0?=w614:bool)
                n188 = case shown="True" w614 {
                  tunnel: w615 -> [w638 w644]
                  tunnel: [w637 w640] -> w613
                  frame False {
                    n189 = Array Subset(array=w638, length=3) -> (w637:dbl[])  [unwired: 1 in]
                  }
                  frame True {
                    n190 = Index Array(array=w644, index=1) -> (element=w648:dbl)
                    n191 = Index Array(array=w644, index=0) -> (element=w647:dbl)
                    n192 = Reciprocal(x=w648) -> (1/x=w642:dbl)
                    n193 = Divide(x=w647, y=w648) -> (x/y=w649:dbl)
                    n194 = Negate(x=w649) -> (-x=w643:dbl)
                    n195 = Build Array(w643, w642, 0.0 ("element")) -> (w640:dbl[])
                  }
                }
                n196 = call "Polybackwards.vi"("Coefficients"=w613, "Y input"=w624) -> ("X output"=w622:dbl)  [unwired: 1 out]
                n197 = Build Array(0.0 ("element"), w622, w621) -> (w619:dbl[])
              }
            }
          }
          frame #3 {
            n198 = Index Array(array=w662, index=1) -> (element=w674:dbl)
            n199 = Index Array(array=w662, index=2) -> (element=w670:dbl)
            n200 = Build Array(w674) -> (w678:dbl[])
            n201 = Index Array(array=w662, index=0) -> (element=w665:dbl)
            n202 = call "2nd_order_Poly_convert.vi"("Calib constants"=w672, "Voltage"=w678) -> ("Eng Values"=w677:dbl[])  [unwired: 4 out]
            n203 = Not A Number/Path/Refnum?(number/path/refnum=w662) -> (NaN/Path/Refnum?=w661:bool[])
            n204 = Or Array Elements(Boolean array=w661) -> (logical OR=w660:bool)
            n205 = Index Array(array=w677, index=0) -> (element=w671:dbl)
            n206 = case shown="False" w660 {
              tunnel: w672 -> [w691 w692]
              tunnel: w671 -> [w689 _]
              tunnel: w670 -> [w686 _]
              tunnel: [w685 w692] -> w669
              tunnel: w665 -> [w683 _]
              tunnel: [w680 w693] -> w664
              tunnel: w663 -> [w679 w693]
              frame False {
                n207 = Equal To 0?(x=w683) -> (x = 0?=w682:bool)
                n208 = Replace Array Subset(array=w691, new element=w689, index=3) -> (w688:dbl[])
                n209 = Format Into String(format string="Bkgnd Fraction %.4f; ", initial string=w679, w683) -> (resulting string=w681:string)  [unwired: 1 in, 1 out]
                n210 = Replace Array Subset(array=w688, new element=w686, index=4) -> (w685:dbl[])
                n211 = Select(t=w679, s=w682, f=w681) -> (s? t:f=w680:string)
              }
              frame True {
              }
            }
          }
        }
      }
      frame "Bkgnd info from table" {
        n212 = stacked-sequence {
          seq-local: [w713 _] -> [_ w755]
          seq-local: [_ w769] -> [_ _]
          seq-local: [w714 _] -> [_ w770]
          seq-local: [w712 _] -> [_ w747]
          tunnel: w711 -> [_ w778]
          tunnel: w710 -> [_ w773]
          tunnel: w709 -> [_ w774]
          tunnel: [_ w778] -> w708
          tunnel: w707 -> [_ w777]
          tunnel: [_ w777] -> w706
          tunnel: [_ w776] -> w705
          tunnel: w704 -> [_ w776]
          tunnel: w703 -> [_ w761]
          tunnel: [_ w751] -> w702
          tunnel: [_ w775] -> w701
          tunnel: w700 -> [_ w775]
          tunnel: [_ "Add FFID Bkgnd Values"] -> w699
          tunnel: [_ TRUE] -> w698
          tunnel: [_ w774] -> w697
          tunnel: w696 -> [_ w757]
          tunnel: [_ w756] -> w695
          frame #0 {
            n213 = while {
              shift-right: [w723] -> _
              shift-left: _ -> [w724]
              shift-right: [w721] -> w714
              shift-left: _ -> [w719]
              shift-right: [w720] -> w713
              shift-left: _ -> [w718]
              shift-right: [w716] -> w712
              shift-left: _ -> [w715]
              stop <- TRUE stop-if-true
              n214 = global read "Meas_global.vi" "Raw data file"() -> (w727:path)
              n215 = Strip Path(path=w727) -> (stripped path=w725:path)  [unwired: 1 out]
              n216 = Build Path(base path=w725, name or relative path="Background_History.xls") -> (appended path=w723:path)
              n217 = Equal?(x=w723, y=w724) -> (x = y?=w722:bool)
              n218 = case shown="False" w722 {
                tunnel: w723 -> [w741 _]
                tunnel: [w734 w744] -> w721
                tunnel: [w731 w743] -> w720
                tunnel: w719 -> [_ w744]
                tunnel: w718 -> [_ w743]
                tunnel: [w728 w742] -> w716
                tunnel: w715 -> [_ w742]
                frame False {
                  n219 = call "Read_File_Simple.vi"("Filename"=w741) -> ("string"=w740:string)  [unwired: 2 in, 7 out]
                  n220 = call "String_to_Ch_names.vi"("Spreadsheet string"=w740) -> ("Ch names"=w730:string[], "String After names"=w737:string)  [unwired: 2 out]
                  n221 = Spreadsheet String To Array(format string="%s", spreadsheet string=w737, array type (2D Dbl)=string[][] []) -> (array=w733:string[][])  [unwired: 1 out]
                  n222 = Search 1D Array(1D array=w730, element="Seconds:since:1st Jan") -> (index of element=w732:i32)  [unwired: 1 out]
                  n223 = Increment(x=w732) -> (x+1=w729:i32)
                  n224 = Index Array(array=w733, index (col)=w732) -> (element=w735:string[])  [unwired: 1 in]
                  n225 = Array Subset(array=w733, index (col)=w729) -> (w731:string[][])  [unwired: 3 in]
                  n226 = Fract/Exp String To Number(string=w735) -> (number=w734:dbl[])  [unwired: 4 out]
                  n227 = Array Subset(array=w730, index=w729) -> (w728:string[])  [unwired: 1 in]
                }
                frame True {
                }
              }
            }
          }
          frame #1 {
            n228 = Unbundle By Name(w774) -> ("Meas start time"=w782:dbl, "Meas end time"=w781:dbl)
            n229 = Decimal String To Number(string=w773) -> (number=w749:i32)  [unwired: 3 out]
            n230 = Format Into String(format string="FF:%d:Bkgnd c^2", w749) -> (resulting string=w748:string)  [unwired: 2 in, 1 out]
            n231 = Search 1D Array(1D array=w747, element=w748) -> (index of element=w746:i32)  [unwired: 1 in]
            n232 = Decrement(x=w749) -> (x-1=w772:i32)
            n233 = Add(x=w782, y=w781) -> (x+y=w780:dbl)
            n234 = Divide(x=w780, y=2.0) -> (x/y=w769:dbl)
            n235 = Index Array(array=w755, index (col)=w772) -> (element=w771:string[])  [unwired: 1 in]
            n236 = Threshold 1D Array(2:w769, 3:w770) -> (0:w754:dbl)  [unwired: 1 out]
            n237 = case shown="1, Default" w746 {
              tunnel: w755 -> [_ w789]
              tunnel: w754 -> [_ w784]
              tunnel: [0.22 w786] -> w750
              tunnel: w746 -> [_ w785]
              frame -1 {
              }
              frame 1, Default {
                n238 = Index Array(array=w789, index (col)=w785) -> (element=w788:string[])  [unwired: 1 in]
                n239 = Fract/Exp String To Number(string=w788) -> (number=w787:dbl[])  [unwired: 4 out]
                n240 = Interpolate 1D Array(1:w784, 2:w787) -> (0:w786:dbl)
              }
            }
            n241 = Fract/Exp String To Number(string=w771) -> (number=w768:dbl[])  [unwired: 4 out]
            n242 = Interpolate 1D Array(1:w754, 2:w768) -> (0:w760:dbl)
            n243 = Build Array(w760) -> (w764:dbl[])
            n244 = Format Into String(format string="Bkgnd Index %.2f; ", initial string=w757, w754) -> (resulting string=w756:string)  [unwired: 1 in, 1 out]
            n245 = call "2nd_order_Poly_convert.vi"("Calib constants"=w761, "Voltage"=w764) -> ("Eng Values"=w763:dbl[])  [unwired: 4 out]
            n246 = Index Array(array=w763, index=0) -> (element=w759:dbl)
            n247 = Replace Array Subset(array=w761, new element=w759, index=3) -> (w752:dbl[])
            n248 = Replace Array Subset(array=w752, new element=w750, index=4) -> (w751:dbl[])
          }
        }
      }
      frame "Add FFID Bkgnd Values" {
        n249 = global read "Plug_in_data_global.vi" "FFID Bkgnd Values"() -> (w794:dbl[])
        n250 = Array Size(array=w794) -> (size(s)=w798:i32)
        n251 = Greater Than 0?(x=w798) -> (x > 0?=w797:bool)
        n252 = case shown="True" w797 {
          tunnel: w796 -> [w806 w820]
          tunnel: [w806 w819] -> w795
          tunnel: w794 -> [_ w810]
          tunnel: w793 -> [w805 w813]
          tunnel: [w805 w807] -> w792
          frame False {
          }
          frame True {
            # "20 blocks of 3 sec bkgnd"
            n253 = Index Array(array=w810, index=1) -> (element=w812:dbl)
            n254 = Index Array(array=w810, index=0) -> (element=w817:dbl)
            n255 = Index Array(array=w810, index=2) -> (element=w809:dbl)
            n256 = Array Subset(array=w810, index=3) -> (w815:dbl[])  [unwired: 1 in]
            n257 = global write "Plug_in_data_global.vi" "FFID Bkgnd Values"(w815) -> ()
            n258 = Replace Array Subset(array=w820, new element=w817, index=3) -> (w819:dbl[])
            n259 = Format Into String(format string="%d blocks of %d Sec Bkgnd; ", initial string=w813, w812, w809) -> (resulting string=w807:string)  [unwired: 1 in, 1 out]
          }
        }
      }
      frame "Add Drift Info" {
        n260 = call "Get_Characters_from_string.vi"("Show Dialog?"=FALSE, "Input string"=w833, "Variable name"="Percentage Drift till Next calibration") -> ("Status"=w840:enum16{"Char in string", "Char not in string"}, "Value"=w841:string)
        n261 = Empty String/Path?(string/path=w829) -> (empty?=w828:bool)
        n262 = case shown="True" w828 {
          tunnel: w829 -> [w874 _]
          tunnel: w823 -> [w872 w876]
          tunnel: [w869 w876] -> w822
          frame False {
            n263 = Unbundle By Name(w872) -> ("Extra Titles"=w873:string[], "Extra Values"=w875:string[])
            n264 = Build Array (concatenate)(w875, w874) -> (w870:string[])
            n265 = Build Array (concatenate)(w873, "Correction:Info" ("string")) -> (w871:string[])
            n266 = Bundle By Name(cluster=w872, "Extra Titles"=w871, "Extra Values"=w870) -> (w869:T1)
          }
          frame True {
          }
        }
        n267 = case shown="\"Char not in string\"" w840 {
          tunnel: [w883 nan ("Value")] -> w832
          tunnel: w841 -> [w879 _]
          frame "Char in string" {
            n268 = Match Pattern(string=w879, regular expression="Drift_Place_Holder") -> (offset past match=w881:i32)  [unwired: 4 out]
            n269 = Greater Than 0?(x=w881) -> (x > 0?=w880:bool)
            n270 = case shown="False" w880 {
              tunnel: [w884 nan ("Value")] -> w883
              tunnel: w879 -> [w885 _]
              frame False {
                n271 = Fract/Exp String To Number(string=w885) -> (number=w884:dbl)  [unwired: 4 out]
              }
              frame True {
              }
            }
          }
          frame "Char not in string" {
          }
        }
        n272 = call "Get_value_from_string.vi"("Show Dialog?"=FALSE, "Input string"=w833, "Variable name"="Minutes Until Next calibration") -> ("Status"=w836:enum16{"Char in string", "Char not in string"}, "Value"=w837:dbl)
        n273 = Array Size(array=w842) -> (size(s)=w843:i32)
        n274 = case shown="\"Char not in string\"" w836 {
          tunnel: [w877 nan ("Value")] -> w831
          tunnel: w837 -> [w877 _]
          frame "Char in string" {
          }
          frame "Char not in string" {
          }
        }
        n275 = Subtract(x=18, y=w843) -> (x-y=w845:i32)
        n276 = Initialize Array(0.0 ("Element Data"), w845) -> (w847:dbl[])
        n277 = Build Array (concatenate)(w842, w847, w832, w831) -> (w827:dbl[])
        n278 = case shown="False" w825 {
          tunnel: w826 -> [w854 _]
          tunnel: w824 -> [w853 _]
          frame False {
            n279 = case shown="\"Psi_eff = f(Umagn.)\", \"Psi_eff, k = f(Umagn.)\"" w853 {
              selector: w853 -> [_ w861 _]
              tunnel: w854 -> [_ w864 _]
              frame "Triangle mesh", "Polynomial surface" {
              }
              frame "Psi_eff = f(Umagn.)", "Psi_eff, k = f(Umagn.)" {
                n280 = Strip Path(path=w864) -> (stripped path=w859:path)  [unwired: 1 out]
                n281 = Build Path(base path=w859, name or relative path="XW_Map.txt") -> (appended path=w862:path)
                n282 = Build Path(base path=w859, name or relative path="XW_Map_CALPTS.txt") -> (appended path=w858:path)
                n283 = call "Does_file_exist_(simple).vi"("Pathname"=w862) -> ("exists?"=w857:bool)
                n284 = call "Does_file_exist_(simple).vi"("Pathname"=w858) -> ("exists?"=w856:bool)
                n285 = And(x=w857, y=w856) -> (x .and. y?=w855:bool)
                n286 = case shown="False" w855 {
                  tunnel: w861 -> [_ w866]
                  frame False {
                    n287 = global write "XW_Map_Global.vi" "Map method"(Map_method."Const. Psi_eff (std.)" ("Map method")) -> ()
                  }
                  frame True {
                    n288 = call "XW_Higher_order_Psi_k_PreProc_PN.vi"("Map method"=w866) -> ()  [unwired: 1 in, 1 out]
                  }
                }
              }
              frame "Const. Psi_eff (std.)" {
                n289 = global write "XW_Map_Global.vi" "Map method"(Map_method."Const. Psi_eff (std.)" ("Map method")) -> ()
              }
            }
          }
          frame True {
          }
        }
      }
    }
  }
  "Calib Coeff" <- w21
  "Analysis Info cluster  Out" <- w5
